vi "Get Parameter.vi"(8 "error in (no error)":errorcluster, 11 "result_from_call in":refnum<class "result_from_call.lvclass">) -> (0 "error out":errorcluster, 2 "Data":variant, 3 "result_from_call out":refnum<class "result_from_call.lvclass">)   [LabVIEW 2015, in "result_from_call.lvclass"]
uses:
  result_from_call.lvclass
  result.lvclass
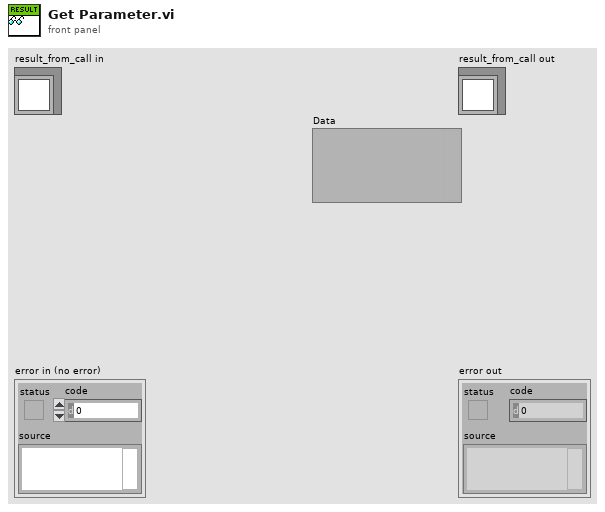
[diagram p1: front panel]
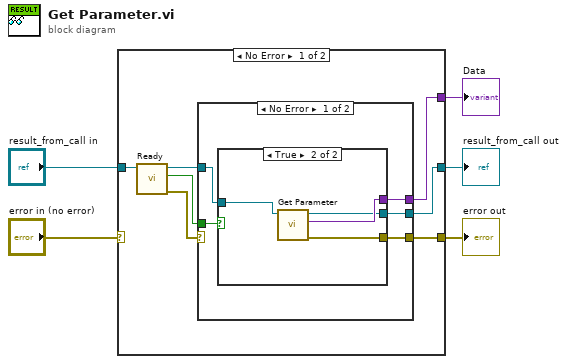
[diagram p0: block diagram]
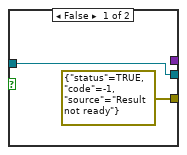
[diagram p2: hidden frame]
diagram:
  n1 = case shown="No Error" "error in (no error)" {
    selector: "error in (no error)" -> [_ w26]
    tunnel: [w12 w26] -> w5
    tunnel: [w11 _] -> w4
    tunnel: "result_from_call in" -> [w10 w27]
    tunnel: [w7 w27] -> w2
    frame No Error {
      n2 = call "Ready.vi"("result_from_call in"=w10) -> ("result_from_call out"=w8:refnum<class "result_from_call.lvclass">, "ready"=w9:bool, "error out"=w6:errorcluster)  [unwired: 7 in]
      n3 = case shown="No Error" w6 {
        selector: w6 -> [_ w25]
        tunnel: [w17 w25] -> w12
        tunnel: [w16 _] -> w11
        tunnel: w9 -> [w15 _]
        tunnel: w8 -> [w14 w24]
        tunnel: [w13 w24] -> w7
        frame No Error {
          n4 = case shown="True" w15 {
            tunnel: [errorcluster {"status"=TRUE, "code"=-1, "source"="Result not ready"} ("error out") w23] -> w17
            tunnel: [_ w22] -> w16
            tunnel: w14 -> [w18 w21]
            tunnel: [w18 w20] -> w13
            frame False {
            }
            frame True {
              n5 = call-parent "Get Parameter.vi"("result in"=w21) -> ("error out"=w23:errorcluster, "Data"=w22:variant, "result out"=w20:refnum<class "result_from_call.lvclass">)  [unwired: 8 in]
            }
          }
        }
        frame Error {
        }
      }
    }
    frame Error {
    }
  }
  "error out" <- w5
  "result_from_call out" <- w2
  "Data" <- w4
